vi "Controllers_PIDZPositionNoWhile-Archived-2024-01-23.vi"(0 "Task In":refnum<k21>, 1 "SP Femto":dbl=0.1, 2 "Loop Time In":i32, 3 "Piezo Offset In / V":dbl format="%.3g", 5 "Error In":errorcluster, 6 "Alpha":dbl=nan format="%.2f", 7 "DC Bias":dbl=0.2, 8 "Beta":dbl=1.0, 9 "PID gains":T1 {"derivative time (Td, min)" format="%.6f"; "integral time (Ti, min)" format="%.6f"; "proportional gain (Kc)" format="%.6f"}, 10 "Iterator In":i32, 11 "Real time Femto / V":dbl=0.10000000000000014) -> (14 "Task Out":refnum<k21>, 15 "Stop?":bool, 16 "Loop Time Out":u32, 17 "Piezo Offset Out / V":dbl format="%.6g", 18 "Runtime / s":dbl, 19 "Error Out":errorcluster)   [LabVIEW 2023]
uses:
  <vilib>/DAQmx/write.llb/DAQmx Write (Analog 1D DBL NChan 1Samp).vi
  <vilib>/addons/control/pid/pid.llb/PID Advanced (DBL).vi
  <vilib>/DAQmx/miscellaneous.llb/DAQmx Fill In Error Info.vi
  <vilib>/addons/control/pid/NI_PID_pid.lvlib
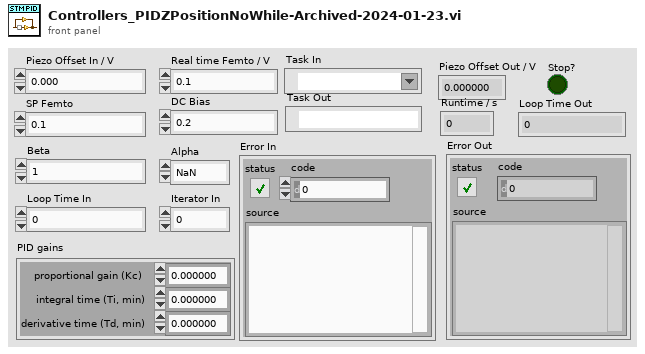
[diagram p1: front panel]
types:
  T1 = cluster{"proportional gain (Kc)":dbl, "integral time (Ti, min)":dbl, "derivative time (Td, min)":dbl}
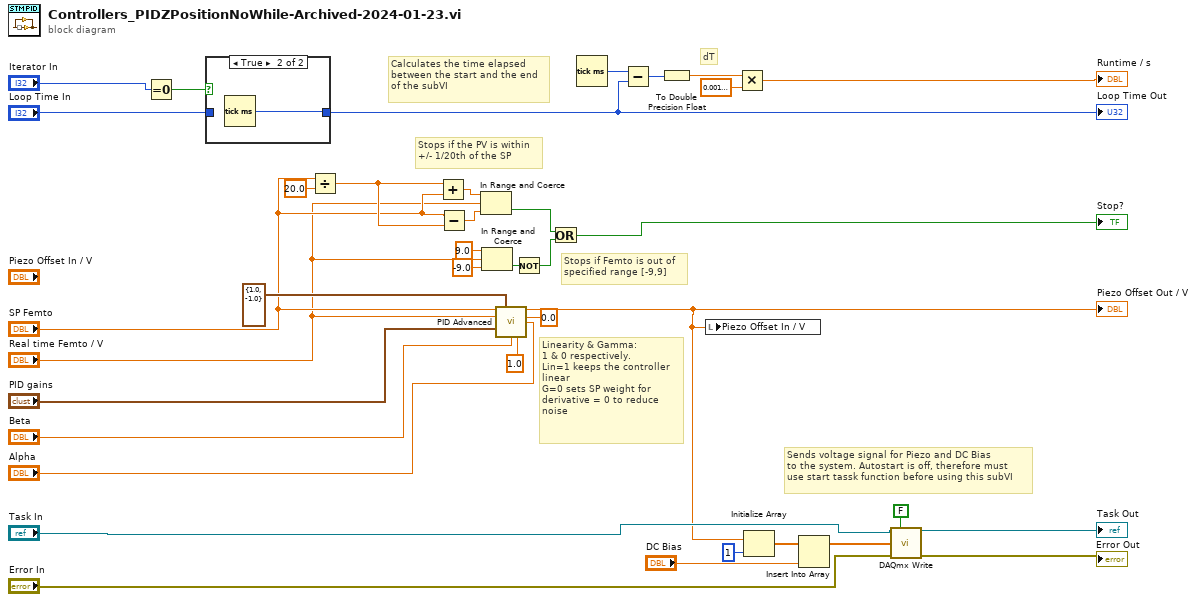
[diagram p0: block diagram]
diagram:
  # "Stops if Femto is out of\nspecified range [-9,9]"
  # "Linearity & Gamma:\n1 & 0 respectively.\nLin=1 keeps the controller \nlinear\nG=0 sets SP weight for \nderivative = 0 to reduce\nnoise"
  # "Calculates the time elapsed\nbetween the start and the end\nof the subVI"
  # "Sends voltage signal for Piezo and DC Bias\nto the system. Autostart is off, therefore must\nuse start tassk function before using this subVI"
  # "Stops if the PV is within\n+/- 1/20th of the SP"
  # "dT"
  n1 = Equal To 0?(x="Iterator In") -> (x = 0?=w4:bool)
  n2 = case shown="True" w4 {
    tunnel: [w38 w39] -> w19
    tunnel: "Loop Time In" -> [w38 _]
    frame False {
    }
    frame True {
      n3 = Tick Count (ms)() -> (millisecond timer value=w39:u32)
    }
  }
  "Loop Time Out" <- w19
  n4 = Divide(x="SP Femto", y=20.0) -> (x/y=w11:dbl)
  n5 = Add(x=w11, y="SP Femto") -> (x+y=w13:dbl)
  n6 = Subtract(x="SP Femto", y=w11) -> (x-y=w12:dbl)
  n7 = In Range and Coerce(upper limit=w13, x="Real time Femto / V", lower limit=w12) -> (In Range?=w6:bool)  [unwired: 1 out]
  n8 = In Range and Coerce(upper limit=9.0, x="Real time Femto / V", lower limit=-9.0) -> (In Range?=w10:bool)  [unwired: 1 out]
  n9 = call-poly <vilib>:"PID Advanced.vi"("setpoint"="SP Femto", "output range"=cluster{"output high":dbl, "output low":dbl} {"output high"=1.0, "output low"=-1.0}, "process variable"="Real time Femto / V", "gamma"=0.0, "alpha"="Alpha", "PID gains"="PID gains", "beta"="Beta", "linearity"=1.0) -> ("output"=w31:dbl)  [unwired: 6 in, 1 out]
  "Piezo Offset Out / V" <- w31
  n10 = Not(x=w10) -> (.not. x?=w7:bool)
  n11 = Or(x=w6, y=w7) -> (x .or. y?=→"Stop?":bool)
  n12 = Tick Count (ms)() -> (millisecond timer value=w20:u32)
  n13 = Subtract(x=w20, y=w19) -> (x-y=w16:u32)
  n14 = To Double Precision Float(number=w16) -> (double precision float=w18:dbl)
  n15 = local write "Piezo Offset In / V"(w31) -> ()
  n16 = Multiply(x=w18, y=0.0010000000474974513) -> (x*y=→"Runtime / s":dbl)
  n17 = Initialize Array(w31, 1 ("dimension size")) -> (w25:dbl[])
  n18 = Insert Into Array(array=w25, new element="DC Bias") -> (w24:dbl[])  [unwired: 1 in]
  n19 = call-poly <vilib>:"DAQmx Write.vi"("task/channels in"="Task In", "auto start"=FALSE, "data"=w24, "error in"="Error In") -> ("task out"=→"Task Out":refnum<k21>, "error out"=→"Error Out":errorcluster)  [unwired: 9 in, 1 out]
